vi "PUBLIC.constructor.vi"(0 "name":string, 2 "data in":string, 5 "error in (no error)":errorcluster) -> (14 "i ref out":refnum<vi>, 16 "data out":string, 19 "error out":errorcluster)   [LabVIEW 2014, in "AG33XXX.lvlib"]
doc: "This is the constructor of a class.\n\nLicense Agreement for this software:\n\nCopyright (C)\nGesellschaft für Schwerionenforschung, GSI\nPlanckstr. 1\n64291 Darmstadt\nGermany\n\nContact: D.Beck@gsi.de \n\nThis program is free software; you can redistribute it and/or modify it under the terms of the \nGNU General Public License as published by the Free Software Foundation; either version 2 of \nthe license, or (at your option) any later version.\n\nThis program is distributed in the hope that it will be useful, but WITHOUT ANY WARRANTY; \nwithout even the implied warranty of MERCHANTABILITY or FITNESS FOR A PARTICULAR PURPOSE. See the GNU General License for more details (http://www.gnu.org).\n\nGesellschaft für Schwerionenforschung, GSI\nPlanckstr. 1, 64291 Darmstadt, Germany\nFor all questions and ideas contact: M.Richter@gsi.de, H.Brand@gsi.de or D.Beck@gsi.de.\nLast update: 16-JUN-2004"
uses:
  AG33XXX.lvlib
  CSCore/CSApplicationBaseClasses/AFGBase/AFGBase.myEventNames.ctl
  CSCore/CSApplicationBaseClasses/DeviceBase/DeviceBase.myEventNames.ctl
  CSCore/CSObj/CSObj.lvlib
  CSCore/BaseProcess/BaseProcess.lvlib
  CSCore/CSSystem/CSSystemLib/CSSystemLib.lvlib
  CSCore/CSApplicationBaseClasses/DeviceBase/DeviceBase.lvlib
  CSCore/CSApplicationBaseClasses/AFGBase/AFGBase.lvlib
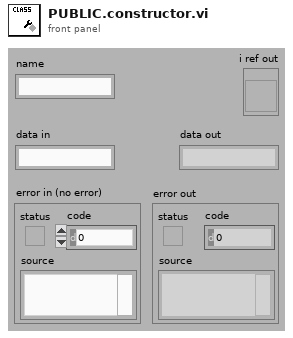
[diagram p1: front panel]
types:
  T1 = enum16{"SetAttribute", "GetAttribute", "CreateAttribute", "DestroyAttribute", "DestroyAllAtributes"}
  T2 = typedef "DeviceBase.lvlib/DeviceBase.myEventNames.ctl" = enum16{"lvmsg://Initialize", "lvmsg://Close", "lvmsg://Configure", "lvmsg://Reset", "lvmsg://IDQuery"}
  T3 = typedef "AFGBase.lvlib/AFGBase.myEventNames.ctl" = enum16{"lvmsg://SetFrequency", "lvmsg://GetFrequency", "lvmsg://SetAmplitude", "lvmsg://GetAmplitude", "lvmsg://SetPhase", "lvmsg://GetPhase", "lvmsg://SetDCOffset", "lvmsg://GetDCOffset", "lvmsg://SetWaveformType", "lvmsg://GetWaveformType", "lvmsg://SetOutputEnabled", "lvmsg://GetOutputEnabled", "lvmsg://SetWaveform", "lvmsg://GetWaveform", "lvmsg://SetTrigger", "lvmsg://GetTrigger", "lvmsg://SetWaveformParams", "lvmsg://GetWaveformParams"}
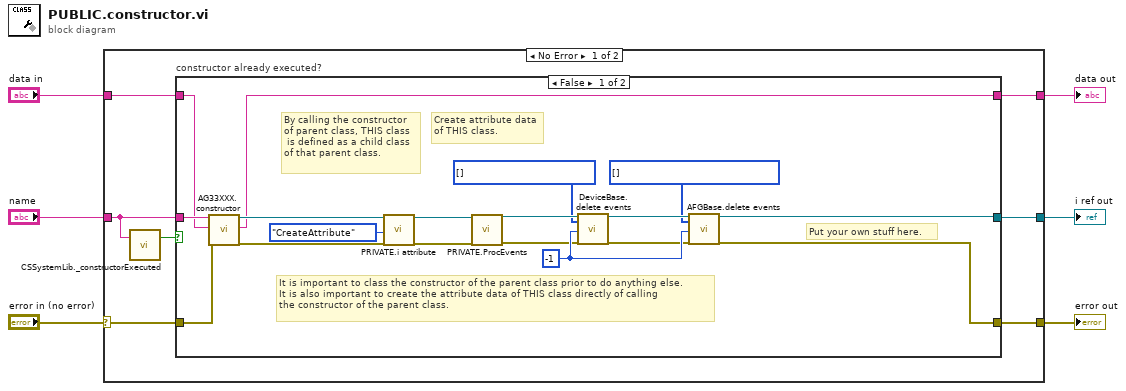
[diagram p0: block diagram]
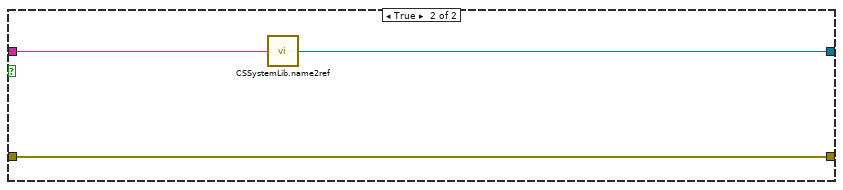
[diagram p2: hidden frame]
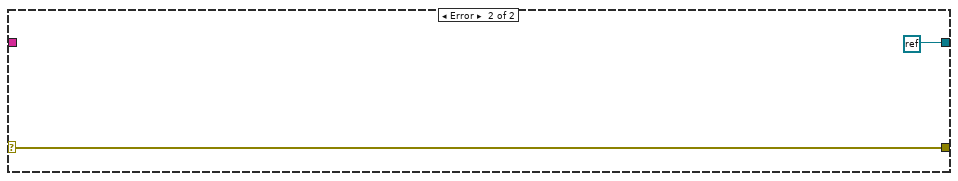
[diagram p3: hidden frame]
diagram:
  n1 = case shown="No Error" "error in (no error)" {
    selector: "error in (no error)" -> [w11 w35]
    tunnel: "name" -> [w10 _]
    tunnel: [w13 refnum<k0> refnum] -> w5
    tunnel: [w12 w35] -> w4
    tunnel: "data in" -> [w8 _]
    tunnel: [w7 _] -> w1
    frame No Error {
      n2 = call "CSSystemLib._constructorExecuted.vi"("name"=w10) -> ("constructor executed?"=w9:bool)  [unwired: 18 in]
      n3 = case "constructor already executed?" shown="False" w9 {
        tunnel: w10 -> [w28 w34]
        tunnel: [w16 w33] -> w13
        tunnel: [w15 w32] -> w12
        tunnel: w11 -> [w25 w32]
        tunnel: w8 -> [w24 _]
        tunnel: [w14 _] -> w7
        frame False {
          w17 = T2[] [] items=["lvmsg://Initialize", "lvmsg://Close", "lvmsg://Configure", "lvmsg://Reset", "lvmsg://IDQuery"]
          w20 = T3[] [] items=["lvmsg://SetFrequency", "lvmsg://GetFrequency", "lvmsg://SetAmplitude", "lvmsg://GetAmplitude", "lvmsg://SetPhase", "lvmsg://GetPhase", "lvmsg://SetDCOffset", "lvmsg://GetDCOffset", "lvmsg://SetWaveformType", "lvmsg://GetWaveformType", "lvmsg://SetOutputEnabled", "lvmsg://GetOutputEnabled", "lvmsg://SetWaveform", "lvmsg://GetWaveform", "lvmsg://SetTrigger", "lvmsg://GetTrigger", "lvmsg://SetWaveformParams", "lvmsg://GetWaveformParams"] ("events")
          w22 = -1 ("ms timeout (10000)")
          # "It is important to class the constructor of the parent class prior to do anything else.\nIt is also important to create the attribute data of THIS class directly of calling\nthe constructor of the parent class."
          # "Put your own stuff here."
          # "Create attribute data\nof THIS class."
          # "By calling the constructor\nof parent class, THIS class\n is defined as a child class\nof that parent class."
          n4 = call "AG33XXX.constructor.vi"("name"=w28, "data in"=w24, "error in (no error)"=w25) -> ("i ref out"=w31:refnum<vi>, "data out"=w14:string, "error out"=w30:errorcluster)  [unwired: 14 in]
          n5 = call "PRIVATE.i attribute.vi"("VI Refnum"=w31, "Action"=T1."CreateAttribute", "error in (no error)"=w30) -> ("VI Refnum out"=w27:refnum<vi>, "error out"=w26:errorcluster)  [unwired: 14 in, 1 out]
          n6 = call "PRIVATE.ProcEvents.vi"("i ref in"=w27, "error in (no error)"=w26) -> ("i ref out"=w19:refnum<vi>, "error out"=w18:errorcluster)  [unwired: 16 in]
          n7 = call "DeviceBase.delete events.vi"("i ref in"=w19, "events"=w17, "ms timeout (10000)"=w22, "error in (no error)"=w18) -> ("i ref out"=w23:refnum<vi>, "error out"=w21:errorcluster)  [unwired: 13 in, 1 out]
          n8 = call "AFGBase.delete events.vi"("i ref in"=w23, "events"=w20, "ms timeout (10000)"=w22, "error in (no error)"=w21) -> ("i ref out"=w16:refnum<vi>, "error out"=w15:errorcluster)  [unwired: 13 in, 1 out]
        }
        frame True {
          n9 = call "CSSystemLib.name2ref.vi"("name"=w34) -> ("obj refnum"=w33:refnum<vi>)
        }
      }
    }
    frame Error {
    }
  }
  "i ref out" <- w5
  "error out" <- w4
  "data out" <- w1
